vi "Kinect Destroy.vi"(8 "error in":errorcluster) -> (0 "error out":errorcluster)   [LabVIEW 2011]
uses:
  Kinect Global Status.vi
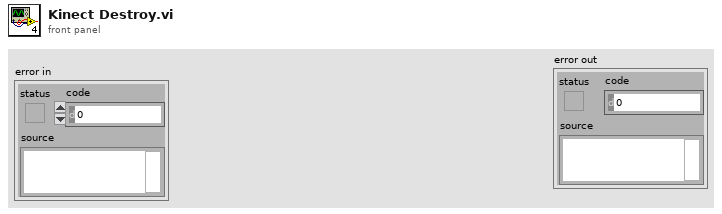
[diagram p1: front panel]
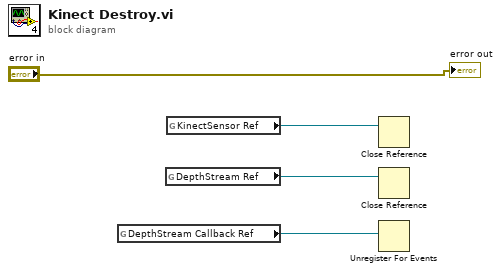
[diagram p0: block diagram]
diagram:
  n1 = global read "Kinect Global Status.vi" "DepthStream Callback Ref"() -> (w3:refnum<k27>)
  n2 = global read "Kinect Global Status.vi" "DepthStream Ref"() -> (w2:refnum<k24>)
  n3 = global read "Kinect Global Status.vi" "KinectSensor Ref"() -> (w1:refnum<k24>)
  n4 = Close Reference(reference=w1) -> ()  [unwired: 1 in, 1 out]
  n5 = Close Reference(reference=w2) -> ()  [unwired: 1 in, 1 out]
  n6 = Unregister For Events(event registration refnum=w3) -> ()  [unwired: 1 in, 1 out]
  "error out" <- "error in"
